vi "Drum Subvi w Notes on Off 2.vi"(5 "Drum Notes On/Off":bool, 8 "Image Dst Out":T1) -> (7 "Red Drum":bool, 9 "Yellow Array":bool[](array[boolean]), 13 "Foot Pedal":bool, 16 "Blue array":bool[](array[boolean]), 17 "Red Array":bool[](array[boolean]), 20 "Green Array":bool[](array[boolean]), 23 "Blue Drum 2":bool, 24 "Yellow Drum":bool, 25 "Green Drum":bool)   [LabVIEW 2009]
uses:
  <vilib>/vision/Image Controls.llb/IMAQ Image.ctl
  <vilib>/Analysis/3filter.llb/Filter Passband Type.ctl
  <vilib>/Analysis/3filter.llb/Butterworth Filter (DBL).vi
  <vilib>/Analysis/NI_AALBase.lvlib
  <vilib>/vision/NI_Vision_Development_Module.lvlib
panel:
  in  "Red Line":T2={"Global Rectangle"=[300, 297, 320, 380], "Contours"=[{"ID"=enum."External", "Type"=2, "Coordinates"=[300, 379, 319, 297]}]} {"Contours"."Type" items=["No Selection", "Point", "Line", "Rectangle", "Oval", "Polygon", "Freehand Region", "Annulus", "Unused2", "Unused3", "Broken Line", "Freehand Line", "Rotated Rectangle"]}
  in  "Blue Line":T2={"Global Rectangle"=[374, 278, 383, 377], "Contours"=[{"ID"=enum."External", "Type"=2, "Coordinates"=[382, 376, 374, 278]}]} {"Contours"."Type" items=["No Selection", "Point", "Line", "Rectangle", "Oval", "Polygon", "Freehand Region", "Annulus", "Unused2", "Unused3", "Broken Line", "Freehand Line", "Rotated Rectangle"]}
  in  "Green Line":T2={"Global Rectangle"=[406, 309, 423, 383], "Contours"=[{"ID"=enum."External", "Type"=2, "Coordinates"=[422, 382, 406, 309]}]} {"Contours"."Type" items=["No Selection", "Point", "Line", "Rectangle", "Oval", "Polygon", "Freehand Region", "Annulus", "Unused2", "Unused3", "Broken Line", "Freehand Line", "Rotated Rectangle"]}
  in  "Yellow Line":T2={"Global Rectangle"=[342, 292, 349, 377], "Contours"=[{"ID"=enum."External", "Type"=2, "Coordinates"=[342, 376, 348, 292]}]} {"Contours"."Type" items=["No Selection", "Point", "Line", "Rectangle", "Oval", "Polygon", "Freehand Region", "Annulus", "Unused2", "Unused3", "Broken Line", "Freehand Line", "Rotated Rectangle"]}
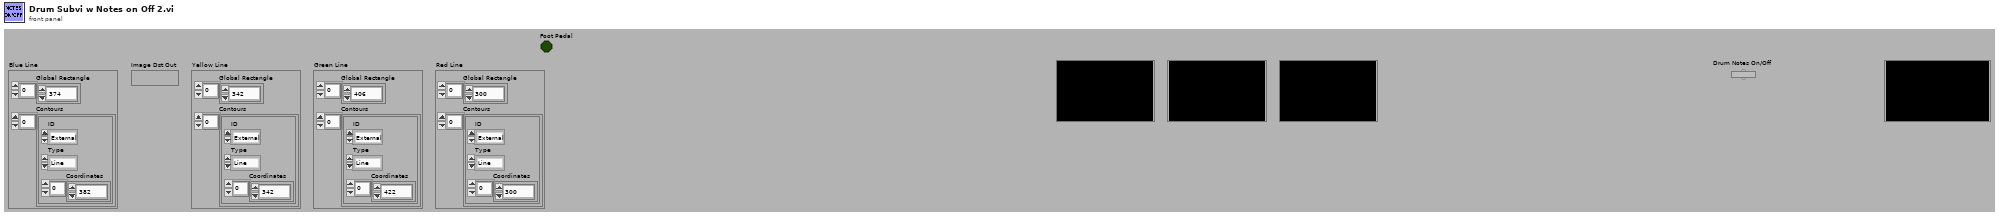
[diagram p1: front panel]
types:
  T1 = typedef "IMAQ Image.ctl" = refnum<image>
  T2 = cluster{"Global Rectangle":i32[], "Contours":cluster{"ID":enum32{"External", "Internal"}, "Type":u32, "Coordinates":i32[]}[]}
  T3 = typedef "NI_AALBase.lvlib/Filter Passband Type.ctl" = enum32{"Lowpass", "Highpass", "Bandpass", "Bandstop"}
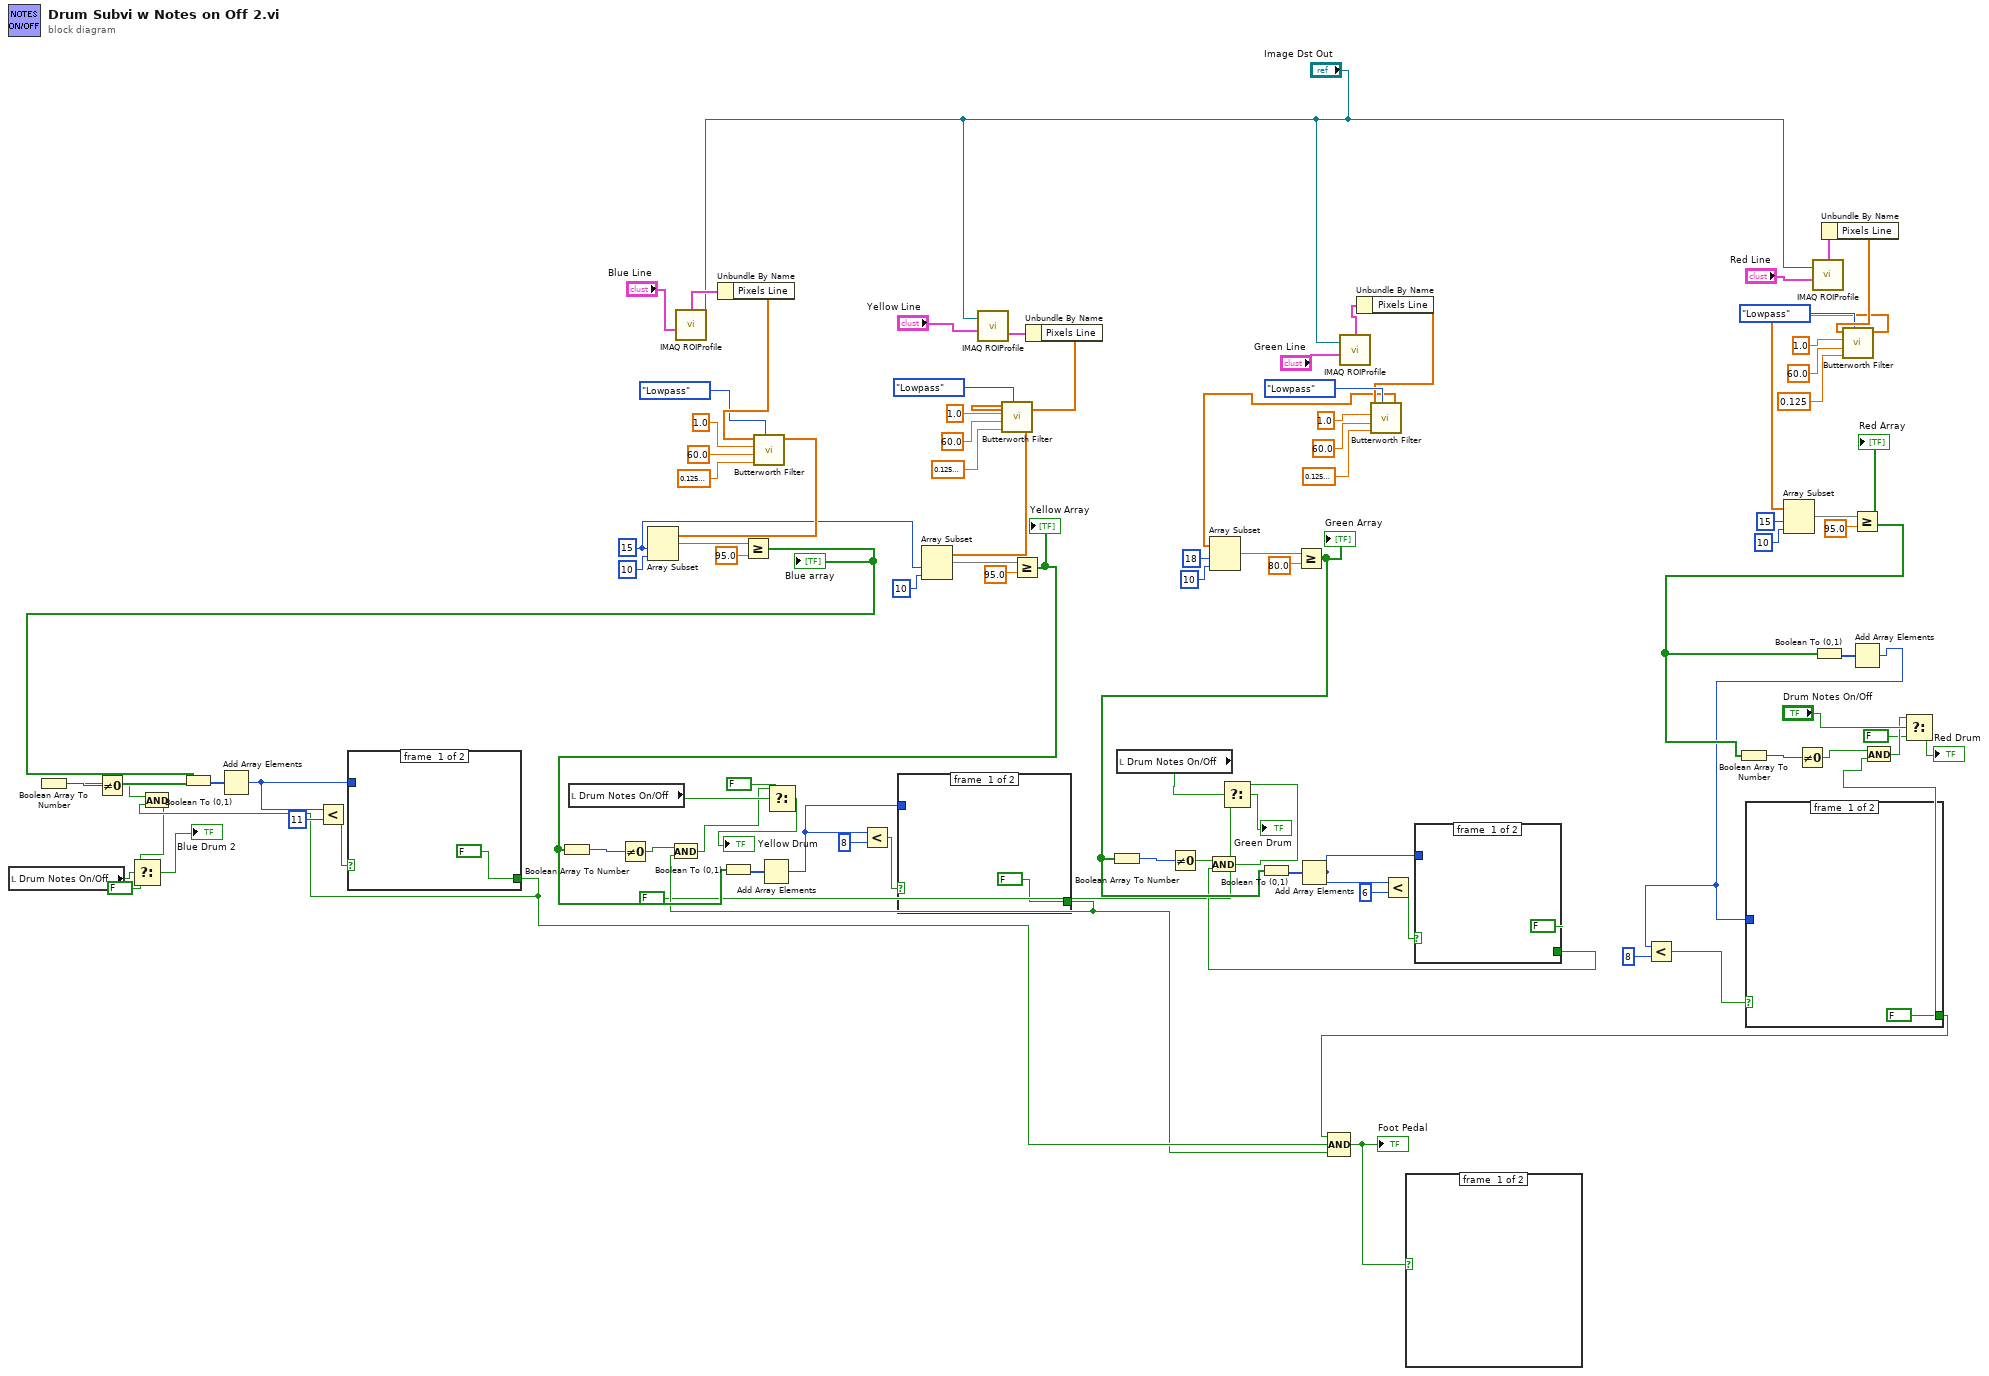
[diagram p0: block diagram]
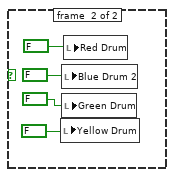
[diagram p2: hidden frame]
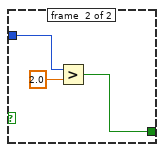
[diagram p3: hidden frame]
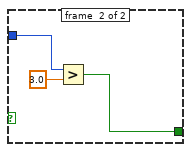
[diagram p4: hidden frame]
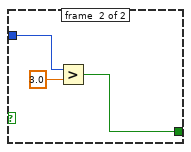
[diagram p5: hidden frame]
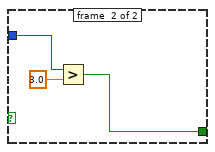
[diagram p6: hidden frame]
diagram:
  w3 = 15 ("index")
  n1 = local read "Drum Notes On/Off"() -> (w19:bool)
  n2 = local read "Drum Notes On/Off"() -> (w20:bool)
  n3 = call "IMAQ ROIProfile"("ROI Descriptor"="Blue Line", "Image"="Image Dst Out") -> ("ROI Graph"=w74:cluster{"x0":sgl, "dx":sgl, "Pixels Line":sgl[]})  [unwired: 1 in, 5 out]
  n4 = Unbundle By Name(w74) -> ("Pixels Line"=w58:sgl[])
  n5 = call-poly <vilib>:"Butterworth Filter.vi"("filter type"=Filter_Passband_Type."Lowpass", "low cutoff freq: fl"=0.12500000000000006 ("low"), "high cutoff freq: fh"=60.0 ("high"), "sampling freq: fs"=1.0 ("sampling"), "X"=w58) -> ("Filtered X"=w84:dbl[])  [unwired: 3 in, 1 out]
  n6 = Array Subset(array=w84, index=w3, length=10) -> (w63:dbl[])
  n7 = Greater Or Equal?(x=w63, y=95.0) -> (x >= y?=w40:bool[])
  "Blue array" <- w40
  n8 = Boolean Array To Number(Boolean array=w40) -> (number=w55:u32)
  n9 = Not Equal To 0?(x=w55) -> (x != 0?=w28:bool)
  n10 = Boolean To (0,1)(Boolean=w40) -> (0, 1=w47:i16[])
  n11 = Add Array Elements(numeric array=w47) -> (sum=w39:i16)
  n12 = Less?(x=w39, y=i16 11) -> (x < y?=w49:bool)
  n13 = case shown="True" w49 {
    tunnel: w39 -> [_ w101]
    tunnel: [FALSE w100] -> w27
    frame #0 {
    }
    frame #1 {
      n14 = Greater?(x=w101, y=3.0) -> (0:w100:bool)
    }
  }
  n15 = And(x=w28, y=w27) -> (x .and. y?=w18:bool)
  n16 = Select(t=w18, s=w19, f=FALSE) -> (s? t:f=→"Blue Drum 2":bool)
  n17 = call "IMAQ ROIProfile"("ROI Descriptor"="Yellow Line", "Image"="Image Dst Out") -> ("ROI Graph"=w71:cluster{"x0":sgl, "dx":sgl, "Pixels Line":sgl[]})  [unwired: 1 in, 5 out]
  n18 = Unbundle By Name(w71) -> ("Pixels Line"=w68:sgl[])
  n19 = call-poly <vilib>:"Butterworth Filter.vi"("filter type"=Filter_Passband_Type."Lowpass", "low cutoff freq: fl"=0.12500000000000006 ("low  2"), "high cutoff freq: fh"=60.0 ("high 2"), "sampling freq: fs"=1.0 ("sampling 2"), "X"=w68) -> ("Filtered X"=w72:dbl[])  [unwired: 3 in, 1 out]
  n20 = Array Subset(array=w72, index=w3, length=10) -> (w65:dbl[])
  n21 = Greater Or Equal?(x=w65, y=95.0) -> (x >= y?=w42:bool[])
  "Yellow Array" <- w42
  n22 = Boolean Array To Number(Boolean array=w42) -> (number=w54:u32)
  n23 = Not Equal To 0?(x=w54) -> (x != 0?=w30:bool)
  n24 = Boolean To (0,1)(Boolean=w42) -> (0, 1=w46:i16[])
  n25 = Add Array Elements(numeric array=w46) -> (sum=w41:i16)
  n26 = Less?(x=w41, y=i16 8) -> (x < y?=w38:bool)
  n27 = case shown="True" w38 {
    tunnel: w41 -> [_ w105]
    tunnel: [FALSE w104] -> w26
    frame #0 {
    }
    frame #1 {
      n28 = Greater?(x=w105, y=3.0) -> (0:w104:bool)
    }
  }
  n29 = And(x=w30, y=w26) -> (x .and. y?=w14:bool)
  n30 = Select(t=w14, s=w20, f=FALSE) -> (s? t:f=→"Yellow Drum":bool)
  n31 = local read "Drum Notes On/Off"() -> (w21:bool)
  n32 = call "IMAQ ROIProfile"("ROI Descriptor"="Green Line", "Image"="Image Dst Out") -> ("ROI Graph"=w75:cluster{"x0":sgl, "dx":sgl, "Pixels Line":sgl[]})  [unwired: 1 in, 5 out]
  n33 = Unbundle By Name(w75) -> ("Pixels Line"=w78:sgl[])
  n34 = call-poly <vilib>:"Butterworth Filter.vi"("filter type"=Filter_Passband_Type."Lowpass", "low cutoff freq: fl"=0.12500000000000006 ("low  3"), "high cutoff freq: fh"=60.0 ("high 3"), "sampling freq: fs"=1.0 ("sampling 3"), "X"=w78) -> ("Filtered X"=w5:dbl[])  [unwired: 3 in, 1 out]
  n35 = Array Subset(array=w5, index=18, length=10) -> (w81:dbl[])
  n36 = Greater Or Equal?(x=w81, y=80.0) -> (x >= y?=w44:bool[])
  "Green Array" <- w44
  n37 = Boolean Array To Number(Boolean array=w44) -> (number=w53:u32)
  n38 = Not Equal To 0?(x=w53) -> (x != 0?=w29:bool)
  n39 = Boolean To (0,1)(Boolean=w44) -> (0, 1=w45:i16[])
  n40 = Add Array Elements(numeric array=w45) -> (sum=w43:i16)
  n41 = Less?(x=w43, y=i16 6) -> (x < y?=w35:bool)
  n42 = case shown="True" w35 {
    tunnel: w43 -> [_ w109]
    tunnel: [FALSE w108] -> w25
    frame #0 {
    }
    frame #1 {
      n43 = Greater?(x=w109, y=2.0) -> (0:w108:bool)
    }
  }
  n44 = And(x=w29, y=w25) -> (x .and. y?=w8:bool)
  n45 = Select(t=w8, s=w21, f=FALSE) -> (s? t:f=→"Green Drum":bool)
  n46 = call "IMAQ ROIProfile"("ROI Descriptor"="Red Line", "Image"="Image Dst Out") -> ("ROI Graph"=w94:cluster{"x0":sgl, "dx":sgl, "Pixels Line":sgl[]})  [unwired: 1 in, 5 out]
  n47 = Unbundle By Name(w94) -> ("Pixels Line"=w91:sgl[])
  n48 = call-poly <vilib>:"Butterworth Filter.vi"("filter type"=Filter_Passband_Type."Lowpass", "low cutoff freq: fl"=0.125 ("low  4"), "high cutoff freq: fh"=60.0 ("high 4"), "sampling freq: fs"=1.0 ("sampling 4"), "X"=w91) -> ("Filtered X"=w23:dbl[])  [unwired: 3 in, 1 out]
  n49 = Array Subset(array=w23, index=15, length=10) -> (w88:dbl[])
  n50 = Greater Or Equal?(x=w88, y=95.0) -> (x >= y?=w32:bool[])
  "Red Array" <- w32
  n51 = Boolean Array To Number(Boolean array=w32) -> (number=w33:u32)
  n52 = Not Equal To 0?(x=w33) -> (x != 0?=w31:bool)
  n53 = Boolean To (0,1)(Boolean=w32) -> (0, 1=w52:i16[])
  n54 = Add Array Elements(numeric array=w52) -> (sum=w4:i16)
  n55 = Less?(x=w4, y=i16 8) -> (x < y?=w50:bool)
  n56 = case shown="True" w50 {
    tunnel: w4 -> [_ w112]
    tunnel: [FALSE w111] -> w34
    frame #0 {
    }
    frame #1 {
      n57 = Greater?(x=w112, y=3.0) -> (0:w111:bool)
    }
  }
  n58 = Compound Arithmetic op=AND(w34, w27, w26) -> (w24:bool)
  "Foot Pedal" <- w24
  n59 = case shown="False" w24 {
    frame #0 {
    }
    frame #1 {
      n60 = local write "Yellow Drum"(FALSE) -> ()
      n61 = local write "Blue Drum 2"(FALSE) -> ()
      n62 = local write "Green Drum"(FALSE) -> ()
      n63 = local write "Red Drum"(FALSE) -> ()
    }
  }
  n64 = And(x=w31, y=w34) -> (x .and. y?=w11:bool)
  n65 = Select(t=w11, s="Drum Notes On/Off", f=FALSE) -> (s? t:f=→"Red Drum":bool)
